vi "PBar-Stop Indeterminate.vi"(0 "VI in":refnum<vi>, 11 "error in (no error)":errorcluster) -> (15 "error out":errorcluster)   [LabVIEW 2020]
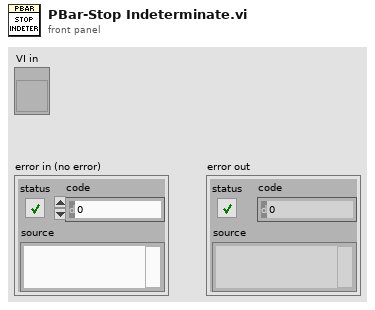
[diagram p1: front panel]
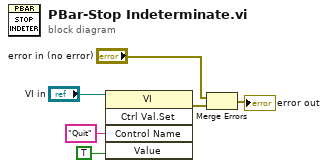
[diagram p0: block diagram]
diagram:
  n1 = invoke class="VI" method="Ctrl Val.Set"(reference="VI in", "Control Name"="Quit", "Value"=TRUE) -> (error out=w1:errorcluster)  [unwired: 2 in, 4 out]
  n2 = Merge Errors("error in (no error)", w1) -> (→"error out":errorcluster)
